vi "test_Basic Deployment.vi"(8 "error in (no error)":errorcluster, 11 "TestCase in":refnum<class "Instrument Addon Error System Tests.lvclass">) -> (0 "error out":errorcluster, 3 "TestCase out":refnum<class "Instrument Addon Error System Tests.lvclass">)   [LabVIEW 2019, in "Instrument Addon Error System Tests.lvclass"]
uses:
  Instrument Addon Error System Tests.lvclass
  <vilib>/addons/_JKI Toolkits/VI Tester/TestCase.llb/TestCase.lvclass
  C:/Program Files (x86)/National Instruments/LabVIEW 2018/vi.lib/addons/_JKI Toolkits/VI Tester/TestCase.llb/TestCase.lvclass
  <vilib>/NI/VeriStand Custom Device Testing Tools/VeriStandTestUtilities/ChassisInformation.ctl
  <vilib>/NI/VeriStand Custom Device Testing Tools/VeriStandTestUtilities/VeriStandTestUtilities.lvlib
  <vilib>/NI/VeriStand Custom Device Testing Tools/VeriStandTestUtilities/TargetInformation.ctl
  <vilib>/NI/VeriStand Custom Device Testing Tools/VeriStandTestUtilities/SystemDefinitionInformation.ctl
panel:
  out "System Definition Information":T1
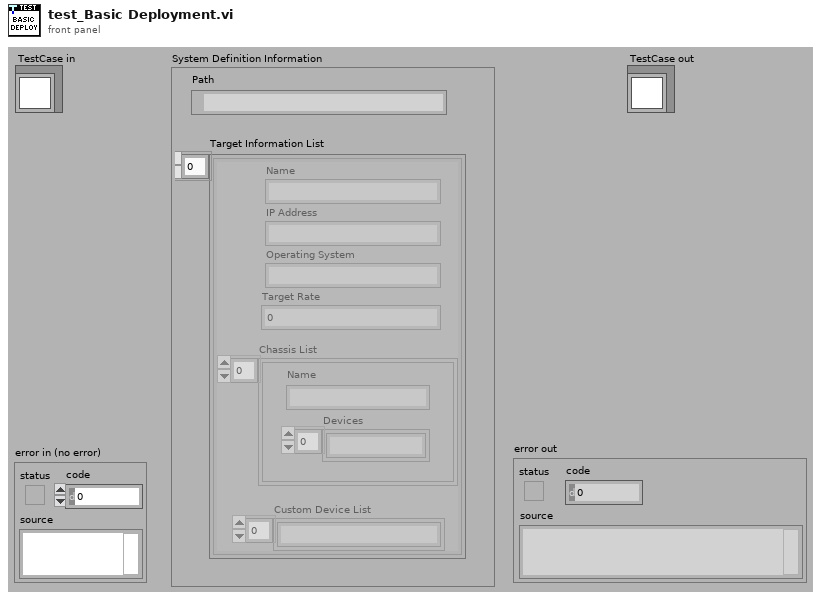
[diagram p1: front panel]
types:
  T1 = typedef "VeriStandTestUtilities.lvlib/SystemDefinitionInformation.ctl" = cluster{"Path":path, "Target Information List":T2[]}
  T2 = typedef "VeriStandTestUtilities.lvlib/TargetInformation.ctl" = cluster{"Name":string, "IP Address":string, "Operating System":string, "Target Rate":dbl, "Chassis List":T3[], "Custom Device List":string[]}
  T3 = typedef "VeriStandTestUtilities.lvlib/ChassisInformation.ctl" = cluster{"Name":string, "Devices":string[]}
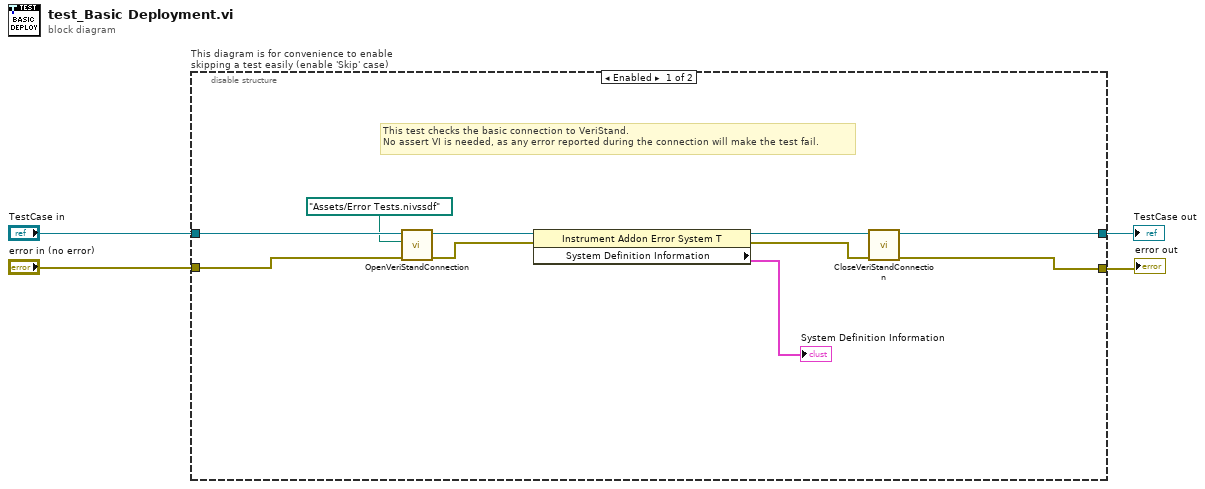
[diagram p0: block diagram]
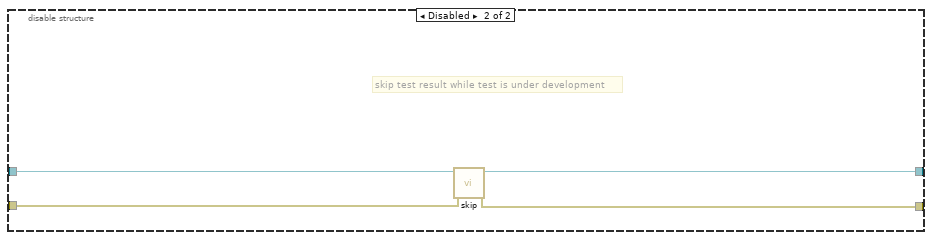
[diagram p2: hidden frame]
diagram:
  n1 = disable-structure "This diagram is for convenience to enable skipping a test easily (enable 'Skip' case)" shown="Enabled" {
    disable-tunnel: "TestCase in" -> [w12 w18]
    disable-tunnel: [w13 w16] -> w1
    disable-tunnel: [w14 w17] -> w3
    disable-tunnel: "error in (no error)" -> [w10 w15]
    frame Enabled {
      # "This test checks the basic connection to VeriStand.\nNo assert VI is needed, as any error reported during the connection will make the test fail."
      n2 = call-dynamic "OpenVeriStandConnection.vi"("error in (no error)"=w10, "System Definition File"=path "Assets/Error Tests.nivssdf", "VeriStand Test Case in"=w12) -> ("error out"=w9:errorcluster, "VeriStand Test Case out"=w11:refnum<class "Instrument Addon Error System Tests.lvclass">)  [unwired: 6 in, 1 out]
      n3 = property class="Instrument Addon Error System T"(reference=w11, error in=w9) -> (reference out=w8:refnum<class "Instrument Addon Error System Tests.lvclass">, error out=w5:errorcluster, "System Definition Information"=→"System Definition Information":T1)
      n4 = call-dynamic "CloseVeriStandConnection.vi"("error in (no error)"=w5, "VeriStand Test Case in"=w8) -> ("error out"=w14:errorcluster, "VeriStand Test Case out"=w13:refnum<class "Instrument Addon Error System Tests.lvclass">)  [unwired: 8 in]
    }
    frame Disabled {
      # "skip test result while test is under development"
      n5 = call <vilib>:"skip.vi"("error in (no error)"=w15, "TestCase in"=w18) -> ("error out"=w17:errorcluster, "TestCase out"=w16:refnum<class "Instrument Addon Error System Tests.lvclass">)  [unwired: 8 in]
    }
  }
  "error out" <- w3
  "TestCase out" <- w1
